vi "string unique values.vi"(7 "index of element":i32, 8 "error in":errorcluster, 11 "sample info":string[][](array[string])) -> (0 "error out":errorcluster, 3 "string array values":string[](array[string]))   [LabVIEW 2016]
doc: "Takes the given value for a string and gives all of the unique values"
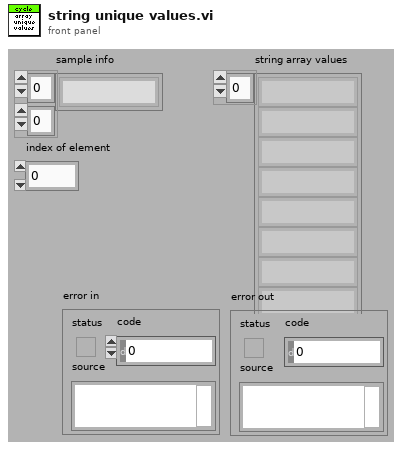
[diagram p1: front panel]
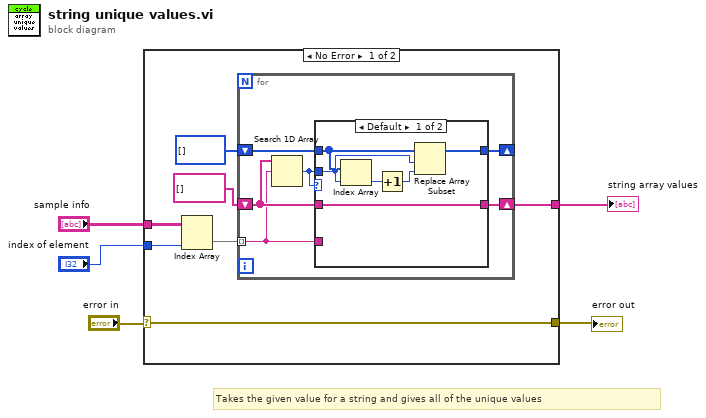
[diagram p0: block diagram]
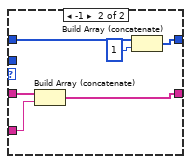
[diagram p2: hidden frame]
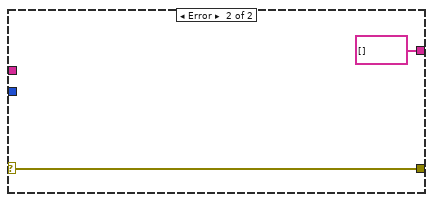
[diagram p3: hidden frame]
diagram:
  # "Takes the given value for a string and gives all of the unique values"
  n1 = case shown="No Error" "error in" {
    selector: "error in" -> [w6 w32]
    tunnel: [w12 string[] []] -> w5
    tunnel: "index of element" -> [w8 _]
    tunnel: "sample info" -> [w7 _]
    tunnel: [w6 w32] -> w1
    frame No Error {
      n2 = Index Array(array=w7, index (col)=w8) -> (element=w11:string[])  [unwired: 1 in]
      n3 = for {
        tunnel: w11 -> [w17] mode=indexing
        shift-right: [w16] -> w12
        shift-left: string[] [] -> [w18]
        shift-right: [w14] -> _
        shift-left: u32[] [] -> [w15]
        n4 = Search 1D Array(1D array=w18, element=w17) -> (index of element=w13:i32)  [unwired: 1 in]
        n5 = case shown="Default" w13 {
          tunnel: w18 -> [w19 w30]
          tunnel: w17 -> [_ w29]
          tunnel: [w19 w28] -> w16
          tunnel: w15 -> [w21 w27]
          tunnel: [w20 w25] -> w14
          tunnel: w13 -> [w24 _]
          frame Default {
            n6 = Index Array(array=w21, index=w24) -> (element=w23:u32)
            n7 = Increment(x=w23) -> (x+1=w22:u32)
            n8 = Replace Array Subset(array=w21, new element=w22, index=w24) -> (w20:u32[])
          }
          frame -1 {
            n9 = Build Array (concatenate)(w30, w29) -> (w28:string[])
            n10 = Build Array (concatenate)(w27, u32 1) -> (w25:u32[])
          }
        }
      }
    }
    frame Error {
    }
  }
  "string array values" <- w5
  "error out" <- w1
